vi "SearchIndex.vi"(8 "error in":errorcluster, 10 "Control Label":string[](array[string]), 11 "UI Ref cluster in":T1) -> (0 "error out":errorcluster, 2 "Index":i32[](array[numeric]), 3 "UI Ref cluster out":T1)   [LabVIEW 2025, in "UI_Library.lvlib" / "UI_Library.lvclass"]
doc: "Get Controls index from label\nIndex = -1 means a Not Available Control Label"
uses:
  UI_Library.lvclass
  Controls/UI_RefCluster.ctl
  <vilib>/Utility/Data Type/Type Definitions/Data Type.ctl
  UI_Library.lvlib
  <vilib>/Utility/Data Type/NI_Data Type.lvlib
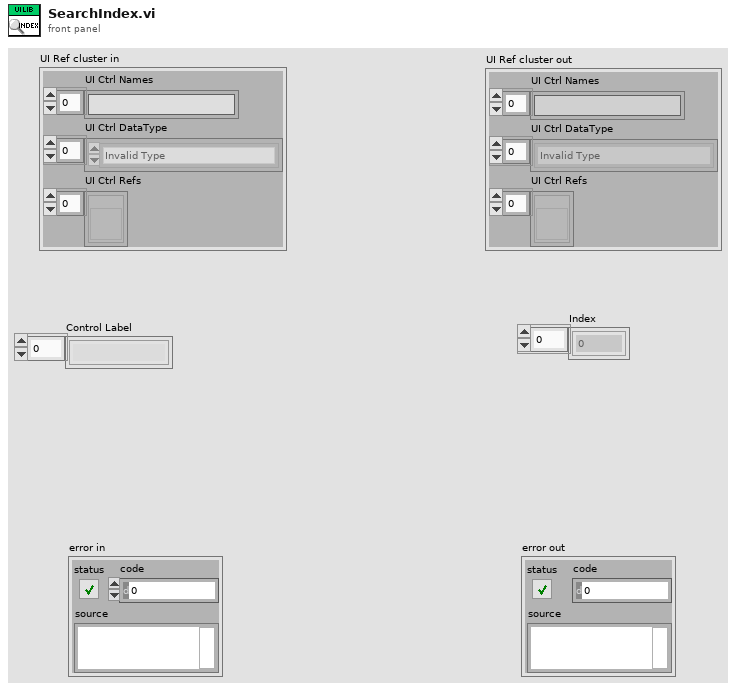
[diagram p1: front panel]
types:
  T1 = typedef "UI_Library.lvlib/UI_RefCluster.ctl" = cluster{"UI Ctrl Names":string[], "UI Ctrl DataType":T2[], "UI Ctrl Refs":refnum<vi>[]}
  T2 = typedef "NI_Data Type.lvlib/Data Type.ctl" = enum8{"Invalid Type", "Void", "I8", "I16", "I32", "I64", "U8", "U16", "U32", "U64", "Single Float", "Double Float", "Extended Float", "Single Complex", "Double Complex", "Extended Complex", "Enum U8", "Enum U16", "Enum U32", "Enum U64", "Single Float With Unit", "Double Float With Unit", "Extended Float With Unit", "Single Complex with Unit", "Double Complex with Unit", "Extended Complex with Unit", "Boolean", "String", "Path", "Picture", "Tag", "Array", "Cluster", "Variant", "LV Variant", "Waveform", "Timestamp", "Digital Waveform", "Digital Data", "ExpressData", "Refnum", "External Data", "VI", "Poly VI", "LabVIEW Class Instance", "Fixed Point", "Set Collection", "Map Collection"}
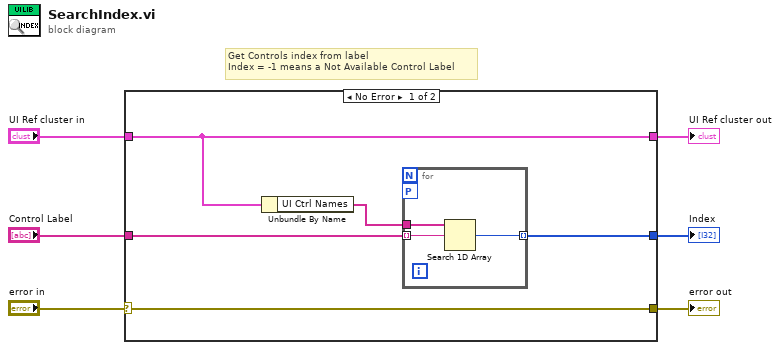
[diagram p0: block diagram]
diagram:
  # "Get Controls index from label\nIndex = -1 means a Not Available Control Label"
  n1 = case shown="No Error" "error in" {
    selector: "error in" -> [w7 w16]
    tunnel: [w7 w16] -> w6
    tunnel: "Control Label" -> [w8 _]
    tunnel: [w10 w15] -> w3
    tunnel: "UI Ref cluster in" -> [w10 w15]
    tunnel: [w9 _] -> w1
    frame No Error {
      n2 = Unbundle By Name(w10) -> ("UI Ctrl Names"=w11:string[])
      n3 = for {
        tunnel: w11 -> [w14]
        tunnel: [w13] -> w9 mode=indexing
        tunnel: w8 -> [w12] mode=indexing
        workers-P: _ -> [_]
        n4 = Search 1D Array(1D array=w14, element=w12) -> (index of element=w13:i32)  [unwired: 1 in]
      }
    }
    frame Error {
    }
  }
  "error out" <- w6
  "UI Ref cluster out" <- w3
  "Index" <- w1
